vi "for2.vi"() -> ()   [LabVIEW 2017]
panel:
  out "最小值":dbl
  out "平均值":dbl
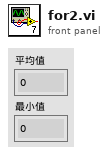
[diagram p1: front panel]
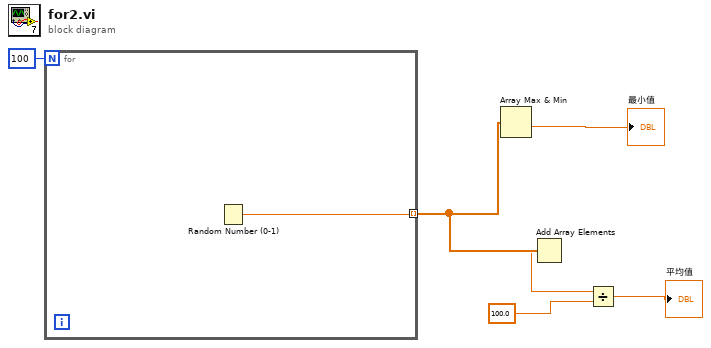
[diagram p0: block diagram]
diagram:
  n1 = for {
    N: 100 -> [_]
    tunnel: [w7] -> w4 mode=indexing
    n2 = Random Number (0-1)() -> (number: 0 to 1=w7:dbl)
  }
  n3 = Array Max & Min(array=w4) -> (min value=→"最小值":dbl)  [unwired: 3 out]
  n4 = Add Array Elements(numeric array=w4) -> (sum=w3:dbl)
  n5 = Divide(x=w3, y=100.0) -> (x/y=→"平均值":dbl)
